vi "Grab Hatch Panel in Auto (BEDPC-GB8-7's conflicted copy 2019-03-16).vi"   [LabVIEW 2018]
uses:
  SubSystems/Hatch Panel Intake/Hatch Panel Intake Global.vi
  SubSystems/Cargo Intake/Cargo Intake Global.vi
  SubSystems/Lift/Lift Global.vi
  SubSystems/Drive Train/Drive Train Global.vi
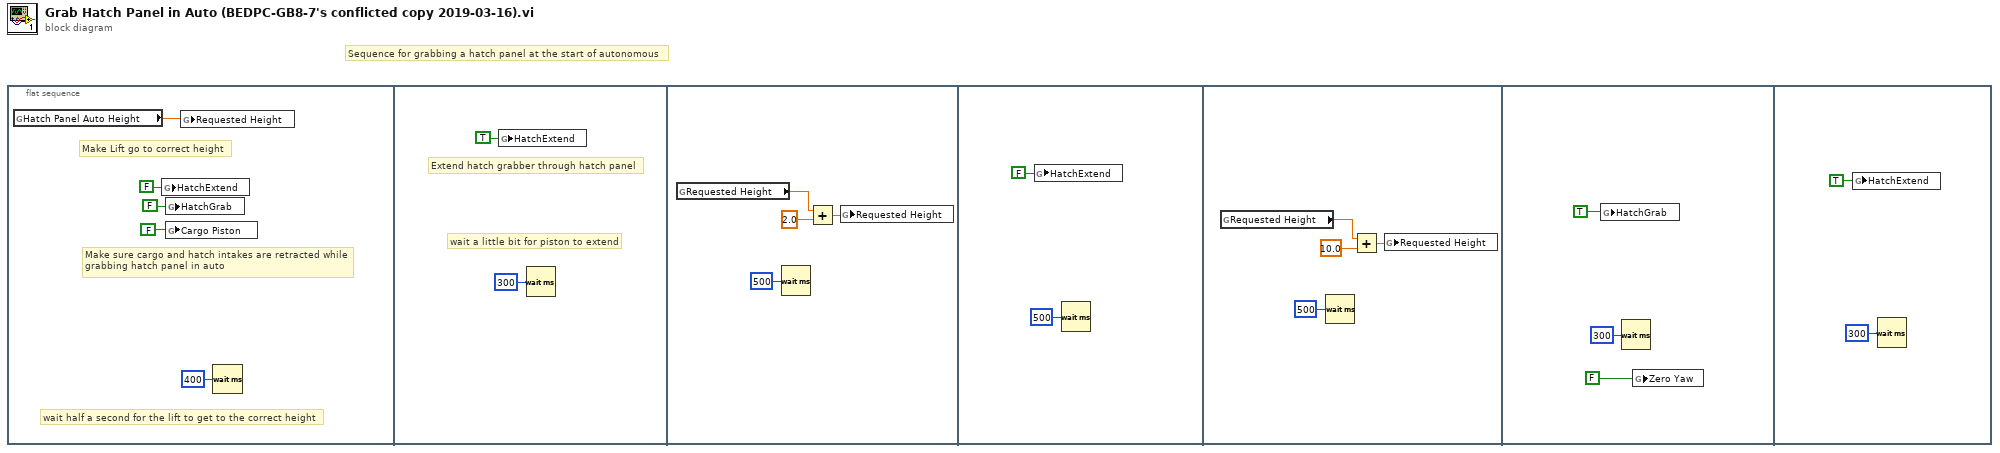
[diagram p0: block diagram]
diagram:
  # "Sequence for grabbing a hatch panel at the start of autonomous"
  n1 = flat-sequence {
    frame #0 {
      # "Make sure cargo and hatch intakes are retracted while\ngrabbing hatch panel in auto"
      # "wait half a second for the lift to get to the correct height"
      # "Make Lift go to correct height"
      n2 = global read "Lift Global.vi" "Hatch Panel Auto Height"() -> (w5:dbl)
      n3 = global write "Hatch Panel Intake Global.vi" "HatchExtend"(FALSE ("HatchExtend")) -> ()
      n4 = global write "Hatch Panel Intake Global.vi" "HatchGrab"(FALSE ("HatchGrab")) -> ()
      n5 = global write "Cargo Intake Global.vi" "Cargo Piston"(FALSE ("Cargo Piston")) -> ()
      n6 = global write "Lift Global.vi" "Requested Height"(w5) -> ()
      n7 = Wait (ms)(milliseconds to wait=u32 400) -> ()  [unwired: 1 out]
    }
    frame #1 {
      # "wait a little bit for piston to extend"
      # "Extend hatch grabber through hatch panel"
      n8 = global write "Hatch Panel Intake Global.vi" "HatchExtend"(TRUE ("HatchExtend")) -> ()
      n9 = Wait (ms)(milliseconds to wait=u32 300) -> ()  [unwired: 1 out]
    }
    frame #2 {
      n10 = global read "Lift Global.vi" "Requested Height"() -> (w9:dbl)
      n11 = Wait (ms)(milliseconds to wait=u32 500) -> ()  [unwired: 1 out]
      n12 = Add(x=w9, y=2.0) -> (x+y=w10:dbl)
      n13 = global write "Lift Global.vi" "Requested Height"(w10) -> ()
    }
    frame #3 {
      n14 = global write "Hatch Panel Intake Global.vi" "HatchExtend"(FALSE ("HatchExtend")) -> ()
      n15 = Wait (ms)(milliseconds to wait=u32 500) -> ()  [unwired: 1 out]
    }
    frame #4 {
      n16 = global read "Lift Global.vi" "Requested Height"() -> (w15:dbl)
      n17 = Wait (ms)(milliseconds to wait=u32 500) -> ()  [unwired: 1 out]
      n18 = Add(x=w15, y=10.0) -> (x+y=w16:dbl)
      n19 = global write "Lift Global.vi" "Requested Height"(w16) -> ()
    }
    frame #5 {
      n20 = global write "Hatch Panel Intake Global.vi" "HatchGrab"(TRUE ("HatchExtend")) -> ()
      n21 = Wait (ms)(milliseconds to wait=u32 300) -> ()  [unwired: 1 out]
      n22 = global write "Drive Train Global.vi" "Zero Yaw"(FALSE ("Reset Field Position")) -> ()
    }
    frame #6 {
      n23 = global write "Hatch Panel Intake Global.vi" "HatchExtend"(TRUE ("HatchExtend")) -> ()
      n24 = Wait (ms)(milliseconds to wait=u32 300) -> ()  [unwired: 1 out]
    }
  }
